vi "Get Client Machine Details.vi"(8 "error in":errorcluster) -> (0 "error out":errorcluster, 1 "ip address":string, 2 "username":string, 3 "hostname":string)   [LabVIEW 2021, in "NI Session Management V1 Client.lvlib" / "Session Reservation.lvclass"]
uses:
  Session Reservation.lvclass
  kernel32.dll
  advapi32.dll
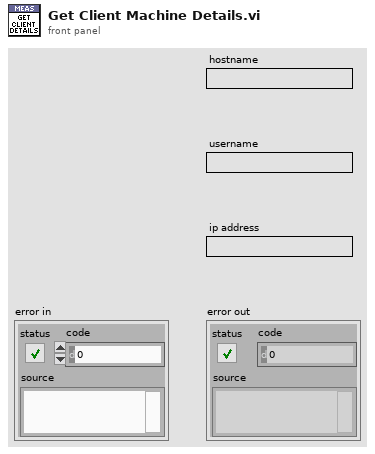
[diagram p1: front panel]
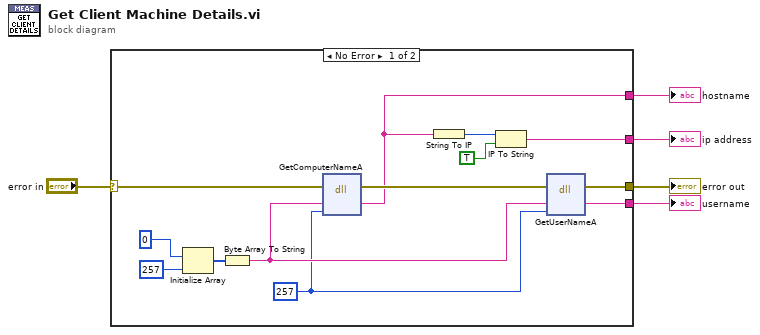
[diagram p0: block diagram]
diagram:
  n1 = case shown="No Error" "error in" {
    selector: "error in" -> [w17 w19]
    tunnel: [w16 _] -> w4
    tunnel: [w15 _] -> w3
    tunnel: [w14 _] -> w2
    tunnel: [w13 w19] -> w1
    frame No Error {
      w7 = u32 257
      n2 = Initialize Array(u8 0, 257 ("dimension size")) -> (w12:u8[])
      n3 = Byte Array To String(unsigned byte array=w12) -> (string=w8:string)
      n4 = dll-call lib="Kernel32.dll" fn="GetComputerNameA"(error in=w17, "lpBuffer"=w8, "lpnSize"=w7) -> (error out=w18:errorcluster, "lpBuffer"=w15:string)  [unwired: 4 in, 1 out]
      n5 = String To IP(1:w15) -> (0:w9:u32)
      n6 = IP To String(1:TRUE ("dot notation? (F)"), 2:w9) -> (0:w16:string)
      n7 = dll-call lib="advapi32.dll" fn="GetUserNameA"(error in=w18, "lpBuffer"=w8, "pcbBuffer"=w7) -> (error out=w13:errorcluster, "lpBuffer"=w14:string)  [unwired: 4 in, 1 out]
    }
    frame Error {
    }
  }
  "ip address" <- w4
  "hostname" <- w3
  "username" <- w2
  "error out" <- w1
